vi "Test MQTT-2.3.1-3.vi"(8 "error in (no error)":errorcluster, 11 "Connection Config":refnum<class "Connection.lvclass">) -> (0 "error out":errorcluster, 3 "Connection Config dup":refnum<class "Connection.lvclass">)   [LabVIEW 2013]
uses:
  <vilib>/LabVIEW Open Source Project/MQTT Connection/MQTT_Connection/Connection/Connection.lvclass
  <vilib>/LabVIEW Open Source Project/MQTT Control Packets/Control Packets/ControlPacket/QualityOfService -- enum.ctl
  <vilib>/LabVIEW Open Source Project/MQTT Control Packets/Control Packets/ControlPacket/Control Packet Type -- enum.ctl
  <vilib>/LabVIEW Open Source Project/MQTT Client/Client class/Client.lvclass/Client.ctl
  <vilib>/LabVIEW Open Source Project/MQTT Control Packets/Control Packets/ControlPacket/ControlPacket.lvclass/ControlPacket.ctl
  <vilib>/addons/_JKI Toolkits/Caraya/classes/Assert/Assert False.vi
  <vilib>/addons/_JKI Toolkits/Caraya/classes/Assert/Assert Not Error.vi
  <vilib>/LabVIEW Open Source Project/MQTT Control Packets/Control Packets/PUBLISH/PUBLISH.lvclass
  <vilib>/addons/_JKI Toolkits/Caraya/classes/Test/Test.lvclass
  <vilib>/LabVIEW Open Source Project/MQTT Control Packets/Control Packets/ControlPacket/ControlPacket.lvclass
  <vilib>/LabVIEW Open Source Project/MQTT Client/Client class/Client.lvclass
  <vilib>/LabVIEW Open Source Project/MQTT Connection/MQTT_Base/Base Class/MQTT_Base.lvclass
  <vilib>/LabVIEW Open Source Project/MQTT Control Packets/Control Packets/CONNECT/CONNECT.lvclass
  <vilib>/LabVIEW Open Source Project/MQTT Control Packets/Control Packets/DISCONNECT/DISCONNECT.lvclass
  <vilib>/addons/_JKI Toolkits/Caraya/classes/Assert/Assert.lvclass
panel:
  out "puback received":bool
  out "Publish Packet ID received":u16[](array[numeric])
  out "publisher error":errorcluster
  out "timed out":bool
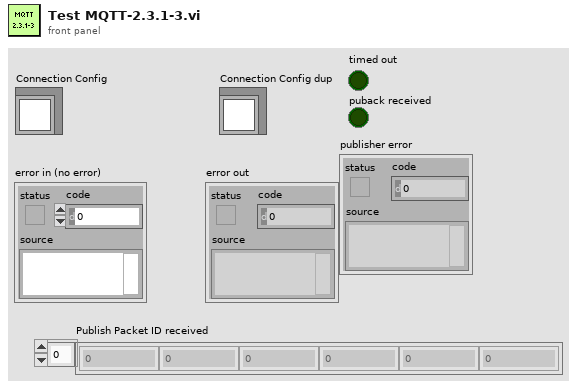
[diagram p1: front panel]
types:
  T1 = typedef "MQTT_Control_Packets.lvlib/ControlPacket.lvclass/Control Packet Type -- enum.ctl" = enum16{"Reserved", "CONNECT", "CONNACK", "PUBLISH", "PUBACK", "PUBREC", "PUBREL", "PUBCOMP", "SUBSCRIBE", "SUBACK", "UNSUBSCRIBE", "UNSUBACK", "PINGREQ", "PINGRESP", "DISCONNECT", "AUTH"}
  T2 = typedef "MQTT_Control_Packets.lvlib/ControlPacket.lvclass/QualityOfService -- enum.ctl" = enum16{"0 (At Most Once)", "1 (At Least Once)", "2 (Exactly Once)"}
  T3 = typedef "MQTT Client.lvlib/Client.lvclass/Public Events -- cluster.ctl" = cluster{"Connection Status":refnum<user-event>, "Connected":refnum<user-event>, "Application Message":refnum<user-event>}
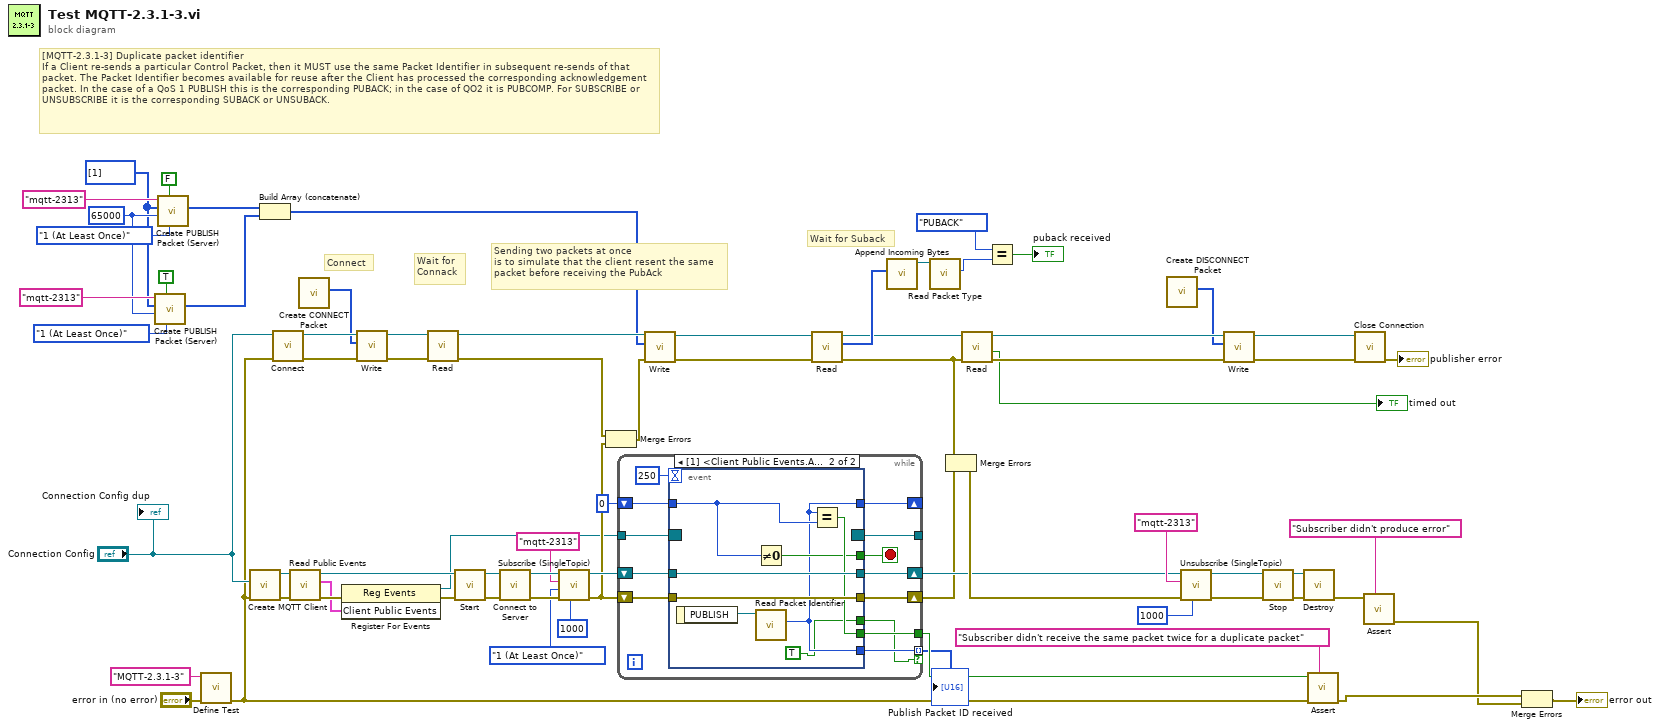
[diagram p0: block diagram]
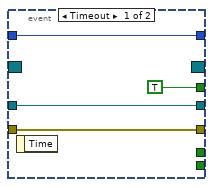
[diagram p2: hidden frame]
diagram:
  w52 = u8[] [1] ("Payload")
  w55 = u16 65000 ("Packet ID (empty: generate new)")
  # "Wait for Suback"
  # "Sending two packets at once\nis to simulate that the client resent the same\npacket before receiving the PubAck"
  # "Wait for\nConnack"
  # "Connect"
  # "[MQTT-2.3.1-3] Duplicate packet identifier\nIf a Client re-sends a particular Control Packet, then it MUST use the same Packet Identifier in subsequent re-sends of that packet. The Packet Identifier becomes available for reuse after the Client has processed the corresponding acknowledgement packet. In the case of a QoS 1 PUBLISH this is the corresponding PUBACK; in the case of QO2 it is PUBCOMP. For SUBSCRIBE or UNSUBSCRIBE it is the corresponding SUBACK or UNSUBACK."
  n1 = call <vilib>:"Create PUBLISH Packet (Server).vi"("QoS"=QualityOfService_--_enum."1 (At Least Once)", "DUP (Re-delivery attempt)"=TRUE, "Packet ID (empty: generate new)"=w55, "Payload"=w52, "Topic Name"="mqtt-2313") -> ("Bytes Stream"=w53:u8[])  [unwired: 3 in, 3 out]
  n2 = call <vilib>:"Create PUBLISH Packet (Server).vi"("QoS"=QualityOfService_--_enum."1 (At Least Once)", "DUP (Re-delivery attempt)"=FALSE, "Packet ID (empty: generate new)"=w55, "Payload"=w52, "Topic Name"="mqtt-2313") -> ("Bytes Stream"=w54:u8[])  [unwired: 3 in, 3 out]
  n3 = call <vilib>:"Define Test.vi"("error in (no error)"="error in (no error)", "Label (VI Title)"="MQTT-2.3.1-3") -> ("error out"=w4:errorcluster)  [unwired: 9 in]
  n4 = call <vilib>:"Create MQTT Client.vi"("error in (no error)"=w4, "Connection Configuration"="Connection Config") -> ("error out"=w18:errorcluster, "Client out"=w20:refnum<class "Client.lvclass">)  [unwired: 8 in]
  n5 = Build Array (concatenate)(w54, w53) -> (w42:u8[])
  n6 = call <vilib>:"Connect.vi"("error in (no error)"=w4, "Connection in"="Connection Config") -> ("error out"=w47:errorcluster, "Connection out"=w50:refnum<class "Connection.lvclass">)  [unwired: 8 in]
  n7 = call <vilib>:"Read Public Events.vi"("error in (no error)"=w18, "Client in"=w20) -> ("error out"=w17:errorcluster, "Client Public Events"=w15:T3, "Client out"=w19:refnum<class "Client.lvclass">)  [unwired: 7 in]
  n8 = call <vilib>:"Create CONNECT Packet.vi"() -> ("Bytes Stream"=w49:u8[])  [unwired: 9 in, 2 out]
  n9 = register-events(error in=w17, w15) -> (reference out=w10:refnum<event-registration>, error out=w16:errorcluster)  [unwired: 1 in]
  n10 = call <vilib>:"Write.vi"("error in (no error)"=w47, "Bytes"=w49, "Connection in"=w50) -> ("error out"=w46:errorcluster, "Connection"=w48:refnum<class "Connection.lvclass">)  [unwired: 7 in]
  n11 = call <vilib>:"Read.vi"("error in (no error)"=w46, "TCPConnection in"=w48) -> ("error out"=w25:errorcluster, "TCPConnection out"=w44:refnum<class "Connection.lvclass">)  [unwired: 5 in, 3 out]
  n12 = call <vilib>:"Start.vi"("error in (no error)"=w16, "MQTT_Base in"=w19) -> ("error out"=w70:errorcluster, "MQTT_Base out"=w71:refnum<class "Client.lvclass">)  [unwired: 7 in, 1 out]
  n13 = call <vilib>:"Connect to Server.vi"("error in (no error)"=w70, "Client in"=w71) -> ("error out"=w67:errorcluster, "Client out"=w68:refnum<class "Client.lvclass">)  [unwired: 6 in, 2 out]
  n14 = call <vilib>:"Subscribe (SingleTopic).vi"("timeout (100ms)"=1000, "error in (no error)"=w67, "QoS"=QualityOfService_--_enum."1 (At Least Once)", "Topic Filter"="mqtt-2313", "MQTT_Base in"=w68) -> ("error out"=w13:errorcluster, "MQTT_Base out"=w14:refnum<class "Client.lvclass">)  [unwired: 4 in, 1 out]
  n15 = Merge Errors(w25, w13) -> (w43:errorcluster)
  n16 = while {
    shift-right: [w81] -> w11
    shift-left: w13 -> [w82]
    shift-right: [w84] -> w12
    shift-left: w14 -> [w83]
    tunnel: w10 -> [w86]
    tunnel: [w85] -> _
    shift-right: [w78] -> _
    shift-left: u16 0 ("Packet Identifier") -> [w77]
    tunnel: [w76] -> w8
    tunnel: [w75] -> w6 mode=indexing if=w74
    stop <- w80 stop-if-true
    n17 = event shown="[1] <Client Public Events.Application Message>: User Event" {
      selector: w86 -> [_ _]
      dyn-events: [_ _] -> w85
      timeout: 250 -> [_ _]
      tunnel: [w90 w98] -> w84
      tunnel: w83 -> [w90 w98]
      tunnel: w82 -> [w89 w97]
      tunnel: [w89 w97] -> w81
      tunnel: [TRUE w93] -> w80
      tunnel: [w87 w92] -> w78
      tunnel: w77 -> [w87 w94]
      tunnel: [_ w95] -> w76
      tunnel: [_ w92] -> w75
      tunnel: [_ TRUE] -> w74
      event Timeout {
        n18 = event-data() -> ()  [unwired: 1 in, 1 out]
      }
      event User Event {
        n19 = event-data() -> ("PUBLISH"=w96:refnum<class "PUBLISH.lvclass">)  [unwired: 1 in]
        n20 = Not Equal To 0?(x=w94) -> (x != 0?=w93:bool)
        n21 = call <vilib>:"Read Packet Identifier.vi"("ControlPacket in"=w96) -> ("Packet Identifier"=w92:u16)  [unwired: 9 in, 1 out]
        n22 = Equal?(x=w92, y=w94) -> (x = y?=w95:bool)
      }
    }
  }
  "Publish Packet ID received" <- w6
  n23 = call <vilib>:"Write.vi"("error in (no error)"=w43, "Bytes"=w42, "Connection in"=w44) -> ("error out"=w40:errorcluster, "Connection"=w41:refnum<class "Connection.lvclass">)  [unwired: 7 in]
  n24 = call <vilib>:"Read.vi"("error in (no error)"=w40, "TCPConnection in"=w41) -> ("error out"=w24:errorcluster, "Bytes"=w39:u8[], "TCPConnection out"=w35:refnum<class "Connection.lvclass">)  [unwired: 5 in, 2 out]
  n25 = call <vilib>:"Append Incoming Bytes.vi"("Incoming Packets"=w39) -> ("ControlPacket"=w38:refnum<class "ControlPacket.lvclass">)  [unwired: 7 in, 3 out]
  n26 = call <vilib>:"Read Packet Type.vi"("ControlPacket in"=w38) -> ("Control Packet Type"=w37:T1)  [unwired: 9 in, 1 out]
  n27 = Merge Errors(w24, w11) -> (w23:errorcluster)
  n28 = call <vilib>:"Read.vi"("error in (no error)"=w24, "TCPConnection in"=w35) -> ("error out"=w33:errorcluster, "timed out"=→"timed out":bool, "TCPConnection out"=w34:refnum<class "Connection.lvclass">)  [unwired: 5 in, 2 out]
  n29 = Equal?(x=Control_Packet_Type_--_enum."PUBACK", y=w37) -> (x = y?=→"puback received":bool)
  n30 = call <vilib>:"Create DISCONNECT Packet.vi"() -> ("Bytes Stream"=w32:u8[])  [unwired: 9 in, 2 out]
  n31 = call <vilib>:"Unsubscribe (SingleTopic).vi"("timeout (100ms)"=1000, "error in (no error)"=w23, "Topic Filter"="mqtt-2313", "MQTT_Base in"=w12) -> ("error out"=w65:errorcluster, "MQTT_Base out"=w66:refnum<class "Client.lvclass">)  [unwired: 5 in, 1 out]
  n32 = call <vilib>:"Write.vi"("error in (no error)"=w33, "Bytes"=w32, "Connection in"=w34) -> ("error out"=w30:errorcluster, "Connection"=w31:refnum<class "Connection.lvclass">)  [unwired: 7 in]
  n33 = call <vilib>:"Stop.vi"("error in (no error)"=w65, "MQTT_Base in"=w66) -> ("error out"=w64:errorcluster, "MQTT_Base out"=w69:refnum<class "Client.lvclass">)  [unwired: 7 in, 1 out]
  n34 = call <vilib>:"Destroy.vi"("error in (no error)"=w64, "MQTT_Base in"=w69) -> ("error out"=w28:errorcluster)  [unwired: 8 in, 1 out]
  n35 = call-poly <vilib>:"Assert.vi"("Label"="Subscriber didn't receive the same packet twice for a duplicate packet", "error in (no error)"=w4, "False?"=w8) -> ("error out"=w3:errorcluster)  [unwired: 8 in]
  n36 = call <vilib>:"Close Connection.vi"("error in (no error)"=w30, "Connection in"=w31) -> ("error out"=→"publisher error":errorcluster)  [unwired: 8 in, 1 out]
  n37 = call-poly <vilib>:"Assert.vi"("Label"="Subscriber didn't produce error", "Not Error?"=w28) -> ("error out"=w2:errorcluster)  [unwired: 9 in]
  n38 = Merge Errors(w3, w2) -> (→"error out":errorcluster)
  "Connection Config dup" <- "Connection Config"
